vi "Calibração.vi"() -> ()   [LabVIEW 2019]
uses:
  <vilib>/Utility/file.llb/Read Delimited Spreadsheet (string).vi
  <vilib>/Utility/file.llb/Write Delimited Spreadsheet (string).vi
panel:
  in  "Valores reserva":T1
  in  "Valores":T1
  in  "Salvar":bool
  in  "Não alterar":bool
  in  "Padrão":bool
  in  "stop":bool
  in  "Iniciar \nCalibração":bool
  out "SHD-PI-01":dbl(knob) scale=0.0..20000.0
  out "SHD-PI-02":dbl
  out "SHD-PI-01":dbl
  out "SHD-PI-02":dbl(knob) scale=0.0..20000.0
  in  "Aferir":bool
  in  "STOP":bool
  # "mmH2O"
  # "mmH2O"
  # "MAX"
  # "MIN"
  # "SHD-PI-01"
  # "mmH2O"
  # "mm"
  # "SHD-PI-02"
  # "mmH2O"
  # "MAX"
  # "MIN"
  # "SHD-PI-01"
  # "mmH2O"
  # "mm"
  # "SHD-PI-02"
  # "KPa"
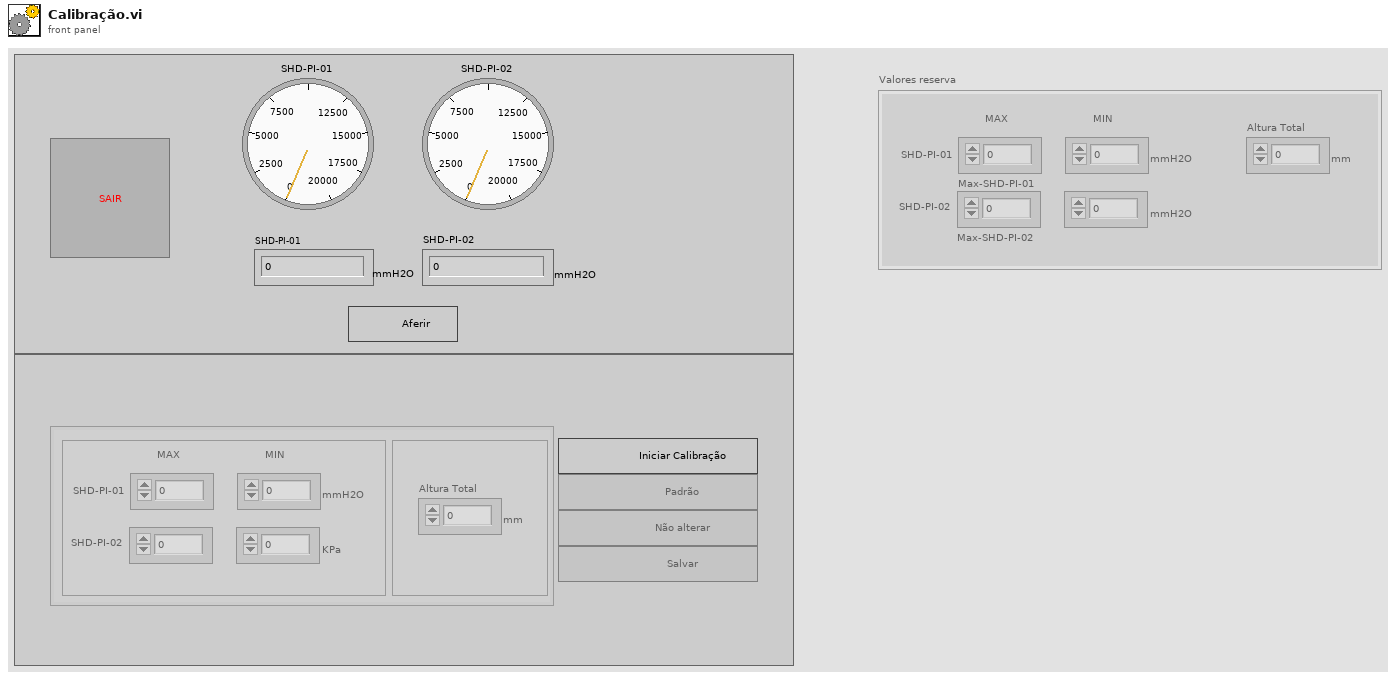
[diagram p1: front panel]
types:
  T1 = cluster{"Max-SHD-PI-01":i32, "Min-SHD-PI-01":i32, "Max-SHD-PI-02":i32, "Min-SHD-PI-02":i32, "Altura Total":i32}
  T2 = enum8{"Enabled", "Disabled", "Disabled and Grayed Out"}
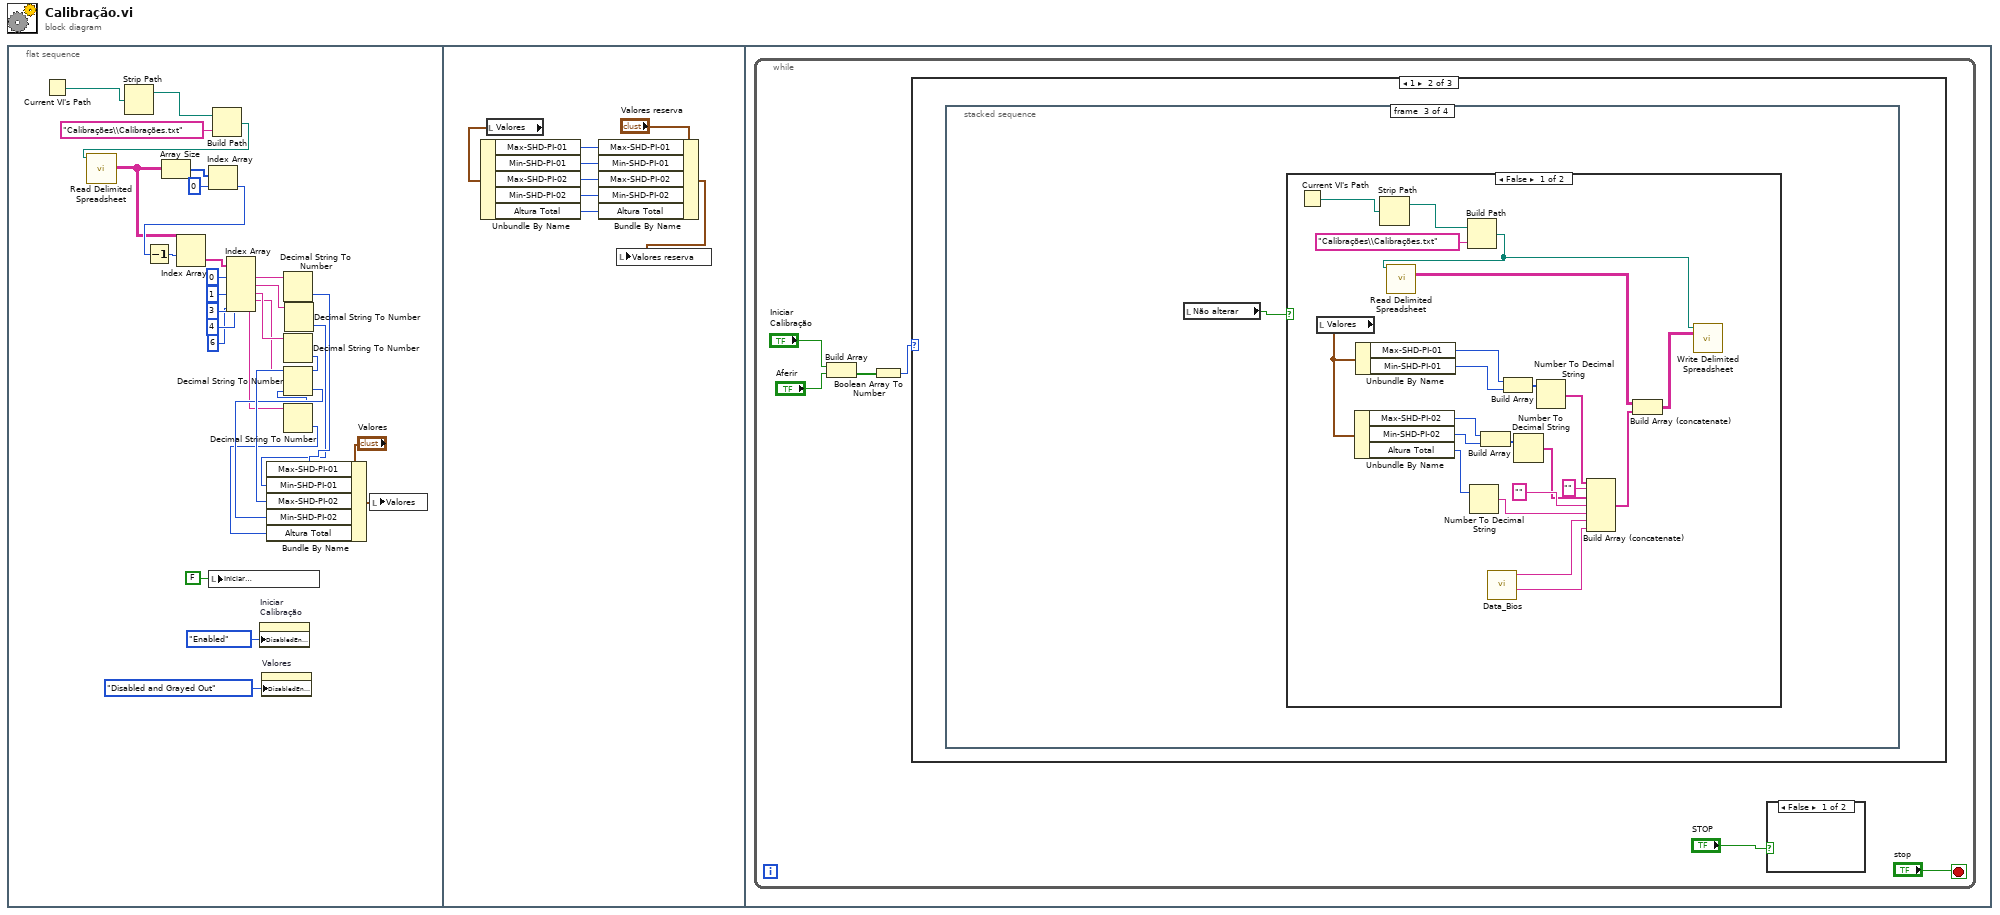
[diagram p0: block diagram]
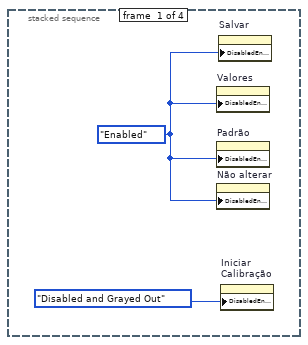
[diagram p3: hidden frame]
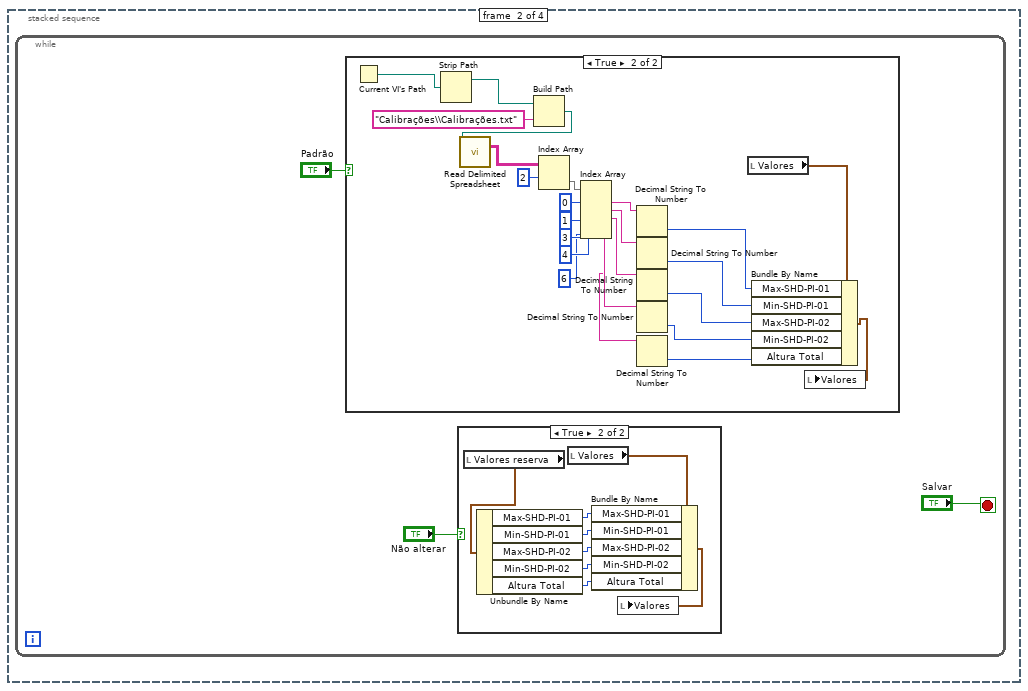
[diagram p4: hidden frame]
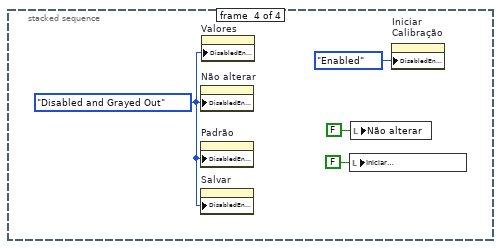
[diagram p8: hidden frame]
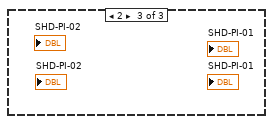
[diagram p9: hidden frame]
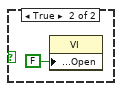
[diagram p10: hidden frame]
diagram:
  n1 = flat-sequence {
    frame #0 {
      n2 = Current VI's Path() -> (path=w4:path)
      n3 = Strip Path(path=w4) -> (stripped path=w3:path)  [unwired: 1 out]
      n4 = local write "Iniciar \nCalibração"(FALSE ("Iniciar \nCalibração")) -> ()
      n5 = Build Path(base path=w3, name or relative path="Calibrações\\Calibrações.txt") -> (appended path=w1:path)
      n6 = call-poly <vilib>:"Read Delimited Spreadsheet.vi"("file path (dialog if empty)"=w1) -> ("all rows"=w9:string[][])  [unwired: 9 in, 5 out]
      n7 = Array Size(array=w9) -> (size(s)=w31:i32[])
      n8 = Index Array(array=w31, index=0) -> (element=w29:i32)
      n9 = Decrement(x=w29) -> (x-1=w28:i32)
      n10 = Index Array(array=w9, index (row)=w28) -> (element=w27:string[])  [unwired: 1 in]
      n11 = Index Array(array=w27, index #1=0 ("index"), index #2=1 ("index"), index #3=3 ("index"), index #4=4 ("index"), index #5=6 ("index")) -> (element #1=w20:string, element #2=w18:string, element #3=w16:string, element #4=w14:string, element #5=w6:string)
      n12 = property on="Iniciar \nCalibração" class="Bool (strict)"("DisabledEnum"=T2."Enabled" ("Disabled")) -> ()  [unwired: 2 in, 2 out]
      n13 = property on="Valores" class="Clust (strict)"("DisabledEnum"=T2."Disabled and Grayed Out" ("Disabled")) -> ()  [unwired: 2 in, 2 out]
      n14 = Decimal String To Number(string=w20) -> (number=w19:i32)  [unwired: 2 in, 1 out]
      n15 = Decimal String To Number(string=w16) -> (number=w15:i32)  [unwired: 2 in, 1 out]
      n16 = Decimal String To Number(string=w6) -> (offset past number=w7:i32, number=w5:i32)  [unwired: 2 in]
      n17 = Decimal String To Number(string=w14, default (0L)=w7) -> (number=w13:i32)  [unwired: 1 in, 1 out]
      n18 = Decimal String To Number(string=w18) -> (number=w17:i32)  [unwired: 2 in, 1 out]
      n19 = Bundle By Name(cluster="Valores", "Max-SHD-PI-01"=w19, "Min-SHD-PI-01"=w17, "Max-SHD-PI-02"=w15, "Min-SHD-PI-02"=w13, "Altura Total"=w5) -> (w21:T1)
      n20 = local write "Valores"(w21) -> ()
    }
    frame #1 {
      n21 = local read "Valores"() -> (w39:T1)
      n22 = Unbundle By Name(w39) -> ("Max-SHD-PI-01"=w38:i32, "Min-SHD-PI-01"=w37:i32, "Max-SHD-PI-02"=w36:i32, "Min-SHD-PI-02"=w35:i32, "Altura Total"=w32:i32)
      n23 = Bundle By Name(cluster="Valores reserva", "Max-SHD-PI-01"=w38, "Min-SHD-PI-01"=w37, "Max-SHD-PI-02"=w36, "Min-SHD-PI-02"=w35, "Altura Total"=w32) -> (w33:T1)
      n24 = local write "Valores reserva"(w33) -> ()
    }
    frame #2 {
      n25 = while {
        stop <- "stop" stop-if-true
        n26 = Build Array("Iniciar \nCalibração", "Aferir") -> (w42:bool[])
        n27 = Boolean Array To Number(Boolean array=w42) -> (number=w41:u32)
        n28 = case shown="1" w41 {
          frame 0, Default {
          }
          frame 1 {
            n29 = stacked-sequence {
              frame #0 {
                w46 = T2."Enabled" ("Disabled")
                n30 = property on="Valores" class="Clust (strict)"("DisabledEnum"=w46) -> ()  [unwired: 2 in, 2 out]
                n31 = property on="Padrão" class="Bool"("DisabledEnum"=w46) -> ()  [unwired: 2 in, 2 out]
                n32 = property on="Não alterar" class="Bool (strict)"("DisabledEnum"=w46) -> ()  [unwired: 2 in, 2 out]
                n33 = property on="Salvar" class="Bool"("DisabledEnum"=w46) -> ()  [unwired: 2 in, 2 out]
                n34 = property on="Iniciar \nCalibração" class="Bool (strict)"("DisabledEnum"=T2."Disabled and Grayed Out" ("Disabled")) -> ()  [unwired: 2 in, 2 out]
              }
              frame #1 {
                n35 = while {
                  stop <- "Salvar" stop-if-true
                  n36 = case shown="True" "Padrão" {
                    frame False {
                    }
                    frame True {
                      n37 = Current VI's Path() -> (path=w54:path)
                      n38 = Strip Path(path=w54) -> (stripped path=w53:path)  [unwired: 1 out]
                      n39 = Build Path(base path=w53, name or relative path="Calibrações\\Calibrações.txt") -> (appended path=w51:path)
                      n40 = call-poly <vilib>:"Read Delimited Spreadsheet.vi"("file path (dialog if empty)"=w51) -> ("all rows"=w72:string[][])  [unwired: 9 in, 5 out]
                      n41 = Index Array(array=w72, index (row)=2) -> (element=w70:string[])  [unwired: 1 in]
                      n42 = Index Array(array=w70, index #1=0 ("index"), index #2=1 ("index"), index #3=3 ("index"), index #4=4 ("index"), index #5=6 ("index")) -> (element #1=w65:string, element #2=w64:string, element #3=w63:string, element #4=w62:string, element #5=w56:string)
                      n43 = Decimal String To Number(string=w65) -> (number=w58:i32)  [unwired: 2 in, 1 out]
                      n44 = Decimal String To Number(string=w64) -> (number=w59:i32)  [unwired: 2 in, 1 out]
                      n45 = Decimal String To Number(string=w63) -> (number=w60:i32)  [unwired: 2 in, 1 out]
                      n46 = Decimal String To Number(string=w62) -> (number=w61:i32)  [unwired: 2 in, 1 out]
                      n47 = Decimal String To Number(string=w56) -> (number=w55:i32)  [unwired: 2 in, 1 out]
                      n48 = local read "Valores"() -> (w74:T1)
                      n49 = Bundle By Name(cluster=w74, "Max-SHD-PI-01"=w58, "Min-SHD-PI-01"=w59, "Max-SHD-PI-02"=w60, "Min-SHD-PI-02"=w61, "Altura Total"=w55) -> (w73:T1)
                      n50 = local write "Valores"(w73) -> ()
                    }
                  }
                  n51 = case shown="True" "Não alterar" {
                    frame False {
                    }
                    frame True {
                      n52 = local read "Valores reserva"() -> (w80:T1)
                      n53 = Unbundle By Name(w80) -> ("Max-SHD-PI-01"=w75:i32, "Min-SHD-PI-01"=w76:i32, "Max-SHD-PI-02"=w77:i32, "Min-SHD-PI-02"=w78:i32, "Altura Total"=w79:i32)
                      n54 = local read "Valores"() -> (w82:T1)
                      n55 = Bundle By Name(cluster=w82, "Max-SHD-PI-01"=w75, "Min-SHD-PI-01"=w76, "Max-SHD-PI-02"=w77, "Min-SHD-PI-02"=w78, "Altura Total"=w79) -> (w81:T1)
                      n56 = local write "Valores"(w81) -> ()
                    }
                  }
                }
              }
              frame #2 {
                n57 = local read "Não alterar"() -> (w83:bool)
                n58 = case shown="False" w83 {
                  frame False {
                    n59 = Current VI's Path() -> (path=w89:path)
                    n60 = local read "Valores"() -> (w100:T1)
                    n61 = Unbundle By Name(w100) -> ("Max-SHD-PI-02"=w98:i32, "Min-SHD-PI-02"=w97:i32, "Altura Total"=w91:i32)
                    n62 = Unbundle By Name(w100) -> ("Max-SHD-PI-01"=w105:i32, "Min-SHD-PI-01"=w104:i32)
                    n63 = Strip Path(path=w89) -> (stripped path=w88:path)  [unwired: 1 out]
                    n64 = Build Path(base path=w88, name or relative path="Calibrações\\Calibrações.txt") -> (appended path=w86:path)
                    n65 = call-poly <vilib>:"Read Delimited Spreadsheet.vi"("file path (dialog if empty)"=w86) -> ("all rows"=w102:string[][])  [unwired: 9 in, 5 out]
                    n66 = Number To Decimal String(number=w91) -> (decimal integer string=w90:string)  [unwired: 1 in]
                    n67 = Build Array(w98, w97) -> (w96:i32[])
                    n68 = call "Data_Bios.vi"() -> ("Hora"=w84:string, "Data"=w85:string)  [unwired: 8 in, 1 out]
                    n69 = Build Array(w105, w104) -> (w103:i32[])
                    n70 = Number To Decimal String(number=w96) -> (decimal integer string=w95:string[])  [unwired: 1 in]
                    n71 = Number To Decimal String(number=w103) -> (decimal integer string=w93:string[])  [unwired: 1 in]
                    n72 = Build Array (concatenate)(w93, "" ("element"), w95, "" ("element"), w90, w85, w84) -> (w92:string[])
                    n73 = Build Array (concatenate)(w102, w92) -> (w101:string[][])
                    n74 = call-poly <vilib>:"Write Delimited Spreadsheet.vi"("file path (dialog if empty)"=w86, "2D data"=w101) -> ()  [unwired: 12 in, 2 out]
                  }
                  frame True {
                  }
                }
              }
              frame #3 {
                w106 = T2."Disabled and Grayed Out" ("Disabled")
                n75 = property on="Não alterar" class="Bool (strict)"("DisabledEnum"=w106) -> ()  [unwired: 2 in, 2 out]
                n76 = property on="Padrão" class="Bool"("DisabledEnum"=w106) -> ()  [unwired: 2 in, 2 out]
                n77 = property on="Salvar" class="Bool"("DisabledEnum"=w106) -> ()  [unwired: 2 in, 2 out]
                n78 = property on="Valores" class="Clust (strict)"("DisabledEnum"=w106) -> ()  [unwired: 2 in, 2 out]
                n79 = local write "Iniciar \nCalibração"(FALSE ("Iniciar \nCalibração")) -> ()
                n80 = local write "Não alterar"(FALSE ("Não alterar")) -> ()
                n81 = property on="Iniciar \nCalibração" class="Bool (strict)"("DisabledEnum"=T2."Enabled" ("Disabled")) -> ()  [unwired: 2 in, 2 out]
              }
            }
          }
          frame 2 {
          }
        }
        n82 = case shown="False" "STOP" {
          frame False {
          }
          frame True {
            n83 = property class="VI"("Front Panel.Open"=FALSE ("Front Panel Window:Open")) -> ()  [unwired: 2 in, 2 out]
          }
        }
      }
    }
  }
